vi "SyncGalvosCamera.vi"(1 "Camera in":refnum<class "Camera.lvclass">, 2 "DAQ in":refnum<class "DAQ.lvclass">, 4 "Return A":dbl=100.0, 5 "error in (no error)":errorcluster, 6 "Scan in":refnum<class "Scan.lvclass">, 7 "Galvo Array":refnum<class "Galvonometer.lvclass">[](array[class])=[refnum, refnum], 8 "Raster":dbl[][](array[numeric])=[[0.0, 0.0], [0.0, 0.0]], 9 "Crop A":dbl=1.0 format="%#_13g", 10 "Settling A":dbl=35.0 format="%#_13g") -> (0 "Sync Err Out":errorcluster, 3 "DAQ out":refnum<class "DAQ.lvclass">)   [LabVIEW 2017]
uses:
  classes/HardwareObjects/DAQ/DAQ.lvclass
  classes/HardwareObjects/Camera/Camera.lvclass
  classes/HardwareObjects/Galvonometer/Galvonometer.lvclass
  classes/Scans/Scan.lvclass
  classes/HardwareObjects/Camera/Camera.lvclass/Camera.ctl
  classes/Scans/Scan.lvclass/Scan.ctl
  classes/HardwareObjects/DAQ/DAQ.lvclass/DAQ.ctl
  classes/HardwareObjects/Galvonometer/Galvonometer.lvclass/Galvonometer.ctl
  classes/HardwareObjects/Galvonometer/Read Max Scan Angle (degrees).vi
  classes/HardwareObjects/Galvonometer/Read Output Scale Factor (V_degrees).vi
  <vilib>/DAQmx/write.llb/DAQmx Write (Analog 2D DBL NChan NSamp).vi
  classes/Scans/Read Total A-scans per frame.vi
  classes/HardwareObjects/Camera/Read Max Frequency (kHz).vi
  classes/HardwareObjects/DAQ/Read Master Counter.vi
  classes/HardwareObjects/DAQ/Read Master Counter Terminal.vi
  classes/HardwareObjects/DAQ/Read Galvo Counter Terminal.vi
  classes/HardwareObjects/DAQ/Read Galvo Counter.vi
  classes/HardwareObjects/DAQ/Read Camera Counter.vi
  classes/HardwareObjects/DAQ/Read Camera Counter Output Terminal.vi
  classes/HardwareObjects/DAQ/Read Galvo Analog Output Channel(s).vi
  classes/HardwareObjects/DAQ/Write Master Counter Task.vi
  classes/HardwareObjects/DAQ/Write Galvo Counter Task.vi
  classes/HardwareObjects/DAQ/Write Galvo Analog Output Task.vi
  classes/HardwareObjects/DAQ/Write Camera Counter Task.vi
  <vilib>/DAQmx/create/channels.llb/DAQmx Create Channel (CO-Pulse Generation-Frequency).vi
  <vilib>/DAQmx/configure/timing.llb/DAQmx Timing (Implicit).vi
  <vilib>/DAQmx/configure/trigger.llb/DAQmx Start Trigger (Digital Edge).vi
  <vilib>/DAQmx/create/channels.llb/DAQmx Create Channel (AO-Voltage-Basic).vi
  <vilib>/DAQmx/configure/timing.llb/DAQmx Timing (Sample Clock).vi
  <vilib>/DAQmx/miscellaneous.llb/DAQmx Fill In Error Info.vi
  <resource>/objmgr/daqmx.rc
panel:
  out "Raster dimensions":i32[](array[numeric])
  out "Active":dbl=300.0
  out "ARC":dbl=500.0
  out "A-scan frequency (Hz)":dbl=125000.0
  out "B-scan frequency":dbl=100.0
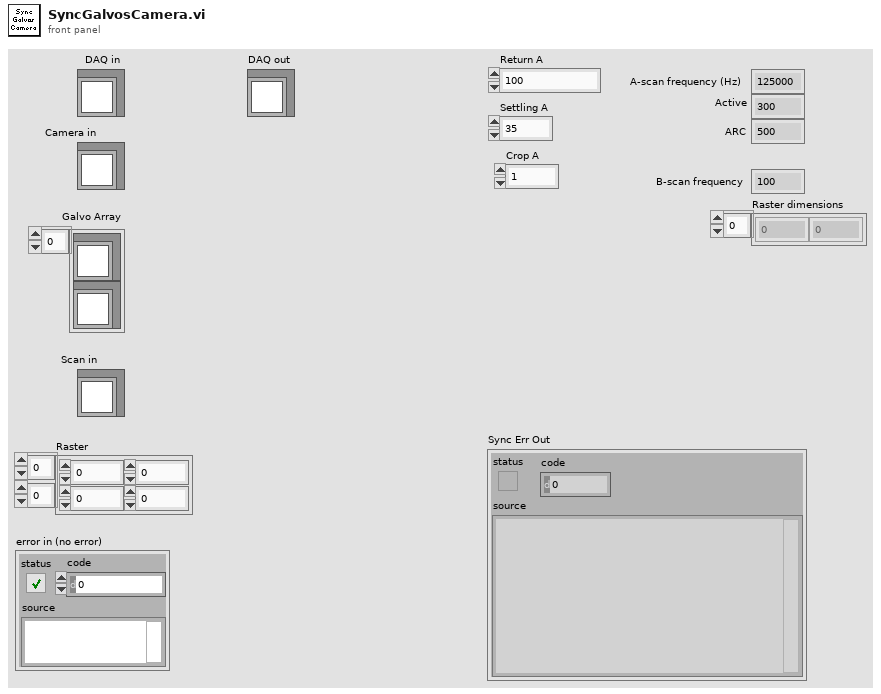
[diagram p1: front panel]
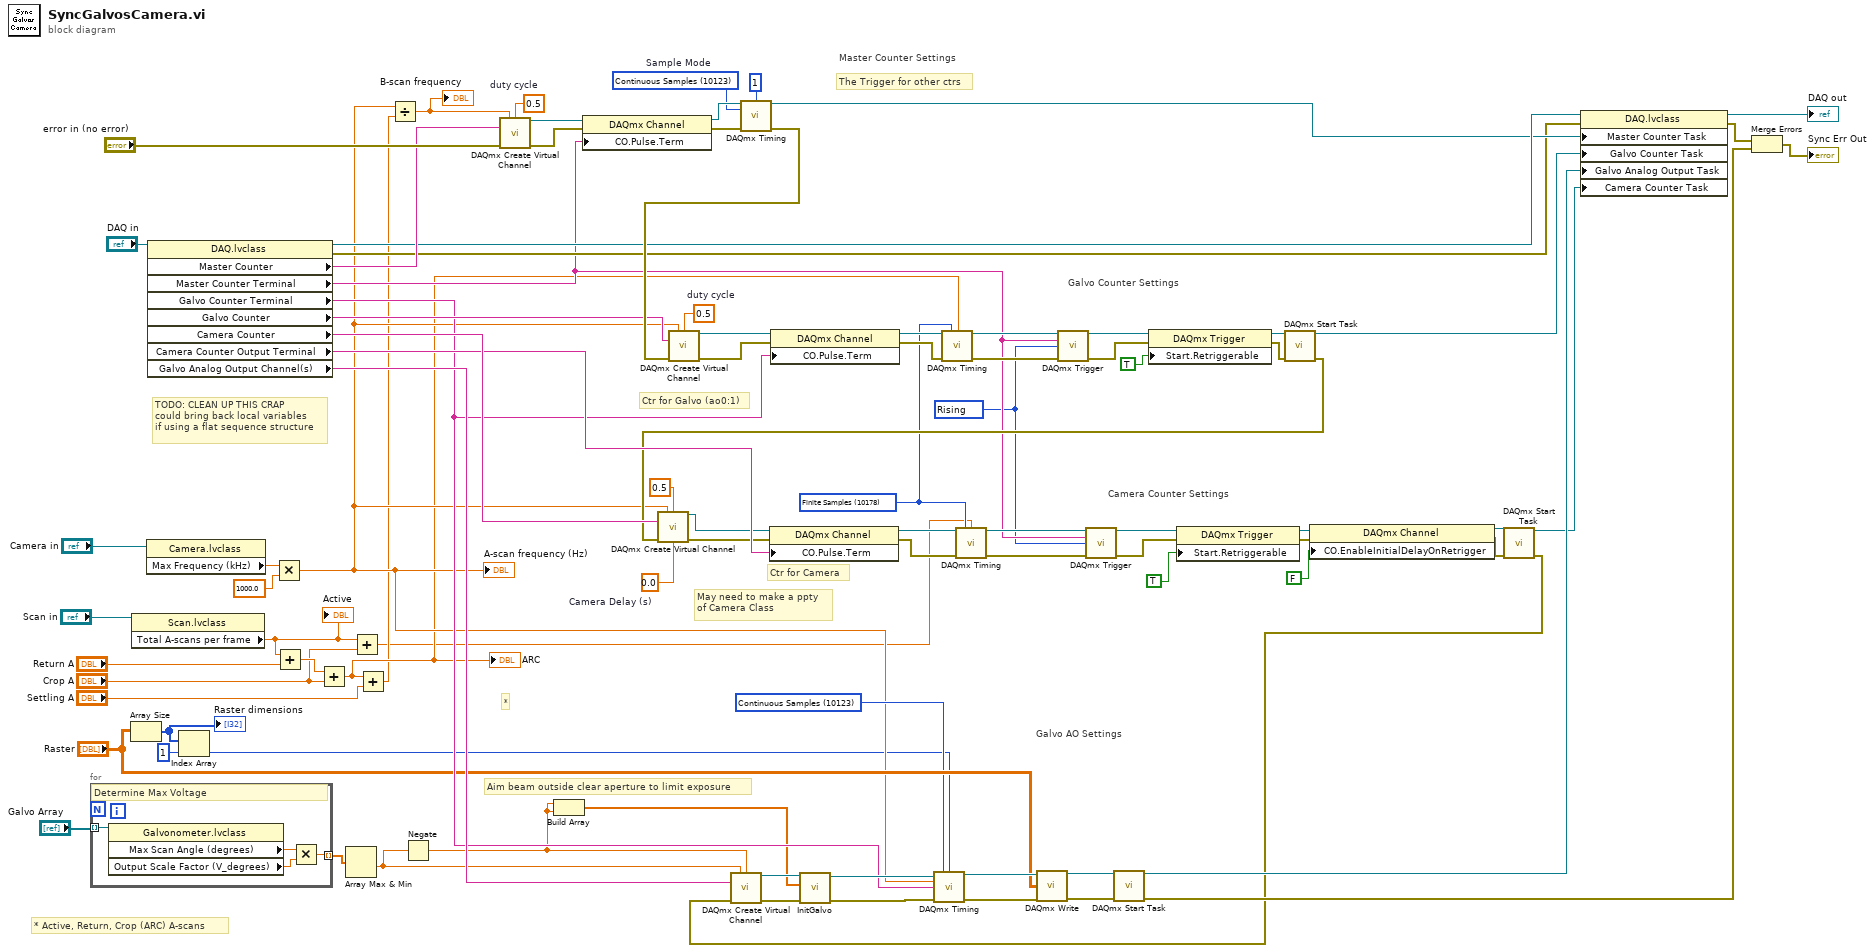
[diagram p0: block diagram]
diagram:
  w11 = 10178 items=["Finite Samples"=10178, "Continuous Samples"=10123, "Hardware Timed Single Point"=12522] ("Sample Mode")
  w26 = 0.0  # Camera Delay (s)
  w16 = 10123 items=["Finite Samples"=10178, "Continuous Samples"=10123, "Hardware Timed Single Point"=12522] ("Sample Mode")
  w74 = 10123 items=["Finite Samples"=10178, "Continuous Samples"=10123, "Hardware Timed Single Point"=12522]  # Sample Mode
  w4 = 10280 items=["Rising"=10280, "Falling"=10171] ("edge")
  w84 = 0.5  # duty cycle
  w89 = 0.5  # duty cycle
  # "Aim beam outside clear aperture to limit exposure"
  # "TODO: CLEAN UP THIS CRAP\ncould bring back local variables\nif using a flat sequence structure"
  # "* Active, Return, Crop (ARC) A-scans"
  # "*"
  # "Camera Counter Settings"
  # "May need to make a ppty\nof Camera Class"
  # "Ctr for Camera"
  # "Galvo AO Settings"
  # "Galvo Counter Settings"
  # "Master Counter Settings"
  # "Ctr for Galvo (ao0:1)"
  # "The Trigger for other ctrs"
  n1 = for {
    tunnel: "Galvo Array" -> [w95] mode=indexing
    tunnel: [w92] -> w46 mode=indexing
    # "Determine Max Voltage"
    n2 = property class="Galvonometer.lvclass"(reference=w95) -> ("Max Scan Angle (degrees)"=w93:dbl, "Output Scale Factor (V_degrees)"=w94:dbl)  [unwired: 1 in, 2 out]
    n3 = Multiply(x=w93, y=w94) -> (x*y=w92:dbl)
  }
  n4 = Array Size(array="Raster") -> (size(s)=w10:i32[])
  "Raster dimensions" <- w10
  n5 = property class="Scan.lvclass"(reference="Scan in") -> ("Total A-scans per frame"=w2:dbl)  [unwired: 1 in, 2 out]
  "Active" <- w2
  n6 = property class="Camera.lvclass"(reference="Camera in") -> ("Max Frequency (kHz)"=w61:sgl)  [unwired: 1 in, 2 out]
  n7 = property class="DAQ.lvclass"(reference="DAQ in") -> (reference out=w56:refnum<class "DAQ.lvclass">, error out=w53:errorcluster, "Master Counter"=w65:tag, "Master Counter Terminal"=w23:tag, "Galvo Counter Terminal"=w19:tag, "Galvo Counter"=w64:tag, "Camera Counter"=w63:tag, "Camera Counter Output Terminal"=w44:tag, "Galvo Analog Output Channel(s)"=w47:tag)  [unwired: 1 in]
  n8 = Index Array(array=w10, index=1) -> (element=w8:i32)
  n9 = Multiply(x=w61, y=1000.0) -> (x*y=w15:dbl)
  "A-scan frequency (Hz)" <- w15
  n10 = Add(x=w2, y="Return A") -> (x+y=w12:dbl)
  n11 = Add(x=w12, y="Crop A") -> (x+y=w7:dbl)
  "ARC" <- w7
  n12 = Array Max & Min(array=w46) -> (min value=w45:dbl)  [unwired: 3 out]
  n13 = Add(x=w2, y="Crop A") -> (x+y=w1:dbl)
  n14 = Add(x=w7, y="Settling A") -> (x+y=w5:dbl)
  n15 = Divide(x=w15, y=w5) -> (x/y=w41:dbl)
  "B-scan frequency" <- w41
  n16 = Negate(x=w45) -> (-x=w14:dbl)
  n17 = call-poly <vilib>:"DAQmx Create Virtual Channel.vi"("frequency"=w41, "duty cycle"=w89, "counter"=w65, "error in"="error in (no error)") -> ("task out"=w91:refnum<k21>, "error out"=w90:errorcluster)  [unwired: 10 in]
  n18 = Build Array(w14, w14) -> (w13:dbl[])
  n19 = property class="DAQmx Channel"(reference=w91, error in=w90, "CO.Pulse.Term"=w23) -> (reference out=w88:refnum<k21>, error out=w87:errorcluster)
  n20 = call-poly <vilib>:"DAQmx Timing.vi"("task/channels in"=w88, "sample mode"=w74, "samples per channel"=1, "error in"=w87) -> ("task out"=w54:refnum<k21>, "error out"=w75:errorcluster)  [unwired: 10 in]
  n21 = call-poly <vilib>:"DAQmx Create Virtual Channel.vi"("frequency"=w15, "duty cycle"=w84, "counter"=w64, "error in"=w75) -> ("task out"=w86:refnum<k21>, "error out"=w85:errorcluster)  [unwired: 10 in]
  n22 = property class="DAQmx Channel"(reference=w86, error in=w85, "CO.Pulse.Term"=w19) -> (reference out=w80:refnum<k21>, error out=w79:errorcluster)
  n23 = call-poly <vilib>:"DAQmx Timing.vi"("task/channels in"=w80, "sample mode"=w11, "samples per channel"=w7, "error in"=w79) -> ("task out"=w78:refnum<k21>, "error out"=w77:errorcluster)  [unwired: 10 in]
  n24 = call-poly <vilib>:"DAQmx Trigger.vi"("task/channels in"=w78, "source"=w23, "edge"=w4, "error in"=w77) -> ("task out"=w82:refnum<k21>, "error out"=w83:errorcluster)  [unwired: 10 in]
  n25 = property class="DAQmx Trigger"(reference=w82, error in=w83, "Start.Retriggerable"=TRUE) -> (reference out=w22:refnum<k21>, error out=w21:errorcluster)
  n26 = call <vilib>:"DAQmx Start Task.vi"("task/channels in"=w22, "error in"=w21) -> ("task out"=w43:refnum<k21>, "error out"=w42:errorcluster)  [unwired: 12 in]
  n27 = call-poly <vilib>:"DAQmx Create Virtual Channel.vi"("frequency"=w15, "duty cycle"=0.5, "counter"=w63, "error in"=w42, "initial delay"=w26) -> ("task out"=w40:refnum<k21>, "error out"=w39:errorcluster)  [unwired: 9 in]
  n28 = property class="DAQmx Channel"(reference=w40, error in=w39, "CO.Pulse.Term"=w44) -> (reference out=w35:refnum<k21>, error out=w34:errorcluster)
  n29 = call-poly <vilib>:"DAQmx Timing.vi"("task/channels in"=w35, "sample mode"=w11, "samples per channel"=w1, "error in"=w34) -> ("task out"=w33:refnum<k21>, "error out"=w32:errorcluster)  [unwired: 10 in]
  n30 = call-poly <vilib>:"DAQmx Trigger.vi"("task/channels in"=w33, "source"=w23, "edge"=w4, "error in"=w32) -> ("task out"=w37:refnum<k21>, "error out"=w38:errorcluster)  [unwired: 10 in]
  n31 = property class="DAQmx Trigger"(reference=w37, error in=w38, "Start.Retriggerable"=TRUE) -> (reference out=w31:refnum<k21>, error out=w30:errorcluster)
  n32 = property class="DAQmx Channel"(reference=w31, error in=w30, "CO.EnableInitialDelayOnRetrigger"=FALSE) -> (reference out=w28:refnum<k21>, error out=w27:errorcluster)
  n33 = call <vilib>:"DAQmx Start Task.vi"("task/channels in"=w28, "error in"=w27) -> ("task out"=w24:refnum<k21>, "error out"=w25:errorcluster)  [unwired: 12 in]
  n34 = call-poly <vilib>:"DAQmx Create Virtual Channel.vi"("maximum value"=w45, "minimum value"=w14, "physical channels"=w47, "error in"=w25) -> ("task out"=w48:refnum<k21>, "error out"=w70:errorcluster)  [unwired: 5 in, 5 out]
  n35 = call "InitGalvo.vi"("error in"=w70, "Output Array"=w13, "task/channels in"=w48) -> ("error out"=w69:errorcluster, "task out"=w68:refnum<k21>)  [unwired: 7 in]
  n36 = call-poly <vilib>:"DAQmx Timing.vi"("task/channels in"=w68, "sample mode"=w16, "samples per channel"=w8, "rate"=w15, "source"=w19, "error in"=w69) -> ("task out"=w71:refnum<k21>, "error out"=w72:errorcluster)  [unwired: 1 in, 7 out]
  n37 = call-poly <vilib>:"DAQmx Write.vi"("task/channels in"=w71, "data"="Raster", "error in"=w72) -> ("task out"=w67:refnum<k21>, "error out"=w66:errorcluster)  [unwired: 1 in, 10 out]
  n38 = call <vilib>:"DAQmx Start Task.vi"("task/channels in"=w67, "error in"=w66) -> ("task out"=w52:refnum<k21>, "error out"=w50:errorcluster)  [unwired: 12 in]
  n39 = property class="DAQ.lvclass"(reference=w56, error in=w53, "Master Counter Task"=w54, "Galvo Counter Task"=w43, "Galvo Analog Output Task"=w52, "Camera Counter Task"=w24) -> (reference out=→"DAQ out":refnum<class "DAQ.lvclass">, error out=w51:errorcluster)
  n40 = Merge Errors(w51, w50) -> (→"Sync Err Out":errorcluster)
